vi "Image position.vi"(7 "pageNum":i32=1, 8 "error in (no error)":errorcluster, 10 "Watermark cluster IN":T1={"Show? (F)"=TRUE, "Watermark type"=enum."Text", "Opacity (%)"=100.0, "Alignment"=enum."Left", "Rotate(°)"=0.0, "Watermark"=enum."Absolute", "X (mm)"=25.0, "Y (mm)"=267.4, "Text"="", "Font"={"Name"="", "Size"=12.0, "Color"=0, "Style"={"Bold"=FALSE, "Italic"=FALSE, "Underline"=FALSE, "Strikeout"=FALSE}}, "Image path"=path "", "Image (%)"=12.0}, 11 "Image IN":refnum<k24>) -> (0 "error out":errorcluster, 2 "output cluster OUT":T1={"Show? (F)"=FALSE, "Watermark type"=enum."Text", "Opacity (%)"=10.0, "Alignment"=enum."Center", "Rotate(°)"=45.0, "Watermark"=enum."Absolute", "X (mm)"=720.0, "Y (mm)"=0.0, "Text"="", "Font"={"Name"="", "Size"=12.0, "Color"=0, "Style"={"Bold"=FALSE, "Italic"=FALSE, "Underline"=FALSE, "Strikeout"=FALSE}}, "Image path"=path "", "Image (%)"=100.0}, 3 "Image OUT":refnum<k24>)   [LabVIEW 2019]
doc: "Version 1.0\nDeveloped by Jean-Marc Simard\nCopyright © 2010, Exaprom Inc.\nAll rights reserved.\nLicense: BSD\n\nWith iTextSharp 4.1.6 (http://itextsharp.sourceforge.net)\nunder Mozilla Public License Version 1.1\n(http://www.mozilla.org/MPL/MPL-1.1.html)"
uses:
  C:/work/niobrara_lv/labview pdf writer fixing/DLL/itextsharp.dll
  DLL/itextsharp.dll
  Controls/Font Controls/Font size.ctl
  Controls/Font Controls/Font color.ctl
  Controls/Font Controls/Font cluster.ctl
  Controls/Header, Footer and Watermark Controls/Header footer horiz alignment.ctl
  <userlib>/Exaprom PDF/Controls/Watermark Page Position.ctl
  Controls/Header, Footer and Watermark Controls/Watermark cluster.ctl
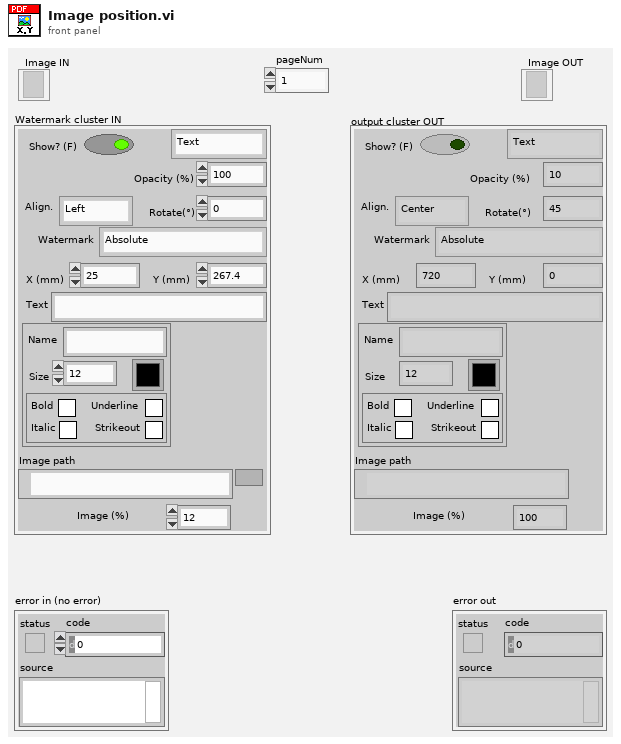
[diagram p1: front panel]
types:
  T1 = typedef "Watermark cluster.ctl" = cluster{"Show? (F)":bool, "Watermark type":enum16{"Text", "Text auto", "Image"}, "Opacity (%)":sgl, "Alignment":T2, "Rotate(°)":sgl, "Watermark":T3, "X (mm)":sgl, "Y (mm)":sgl, "Text":string, "Font":T4, "Image path":path, "Image (%)":sgl}
  T2 = typedef "Header footer horiz alignment.ctl" = enum16{"Left", "Center", "Right"}
  T3 = typedef "Watermark Page Position.ctl" = enum16{"Absolute", "Center on page", "Center on text section"}
  T4 = typedef "Font cluster.ctl" = cluster{"Name":string, "Size":T5, "Color":T6, "Style":cluster{"Bold":bool, "Italic":bool, "Underline":bool, "Strikeout":bool}}
  T5 = typedef "Font size.ctl" = sgl
  T6 = typedef "Font color.ctl" = u32
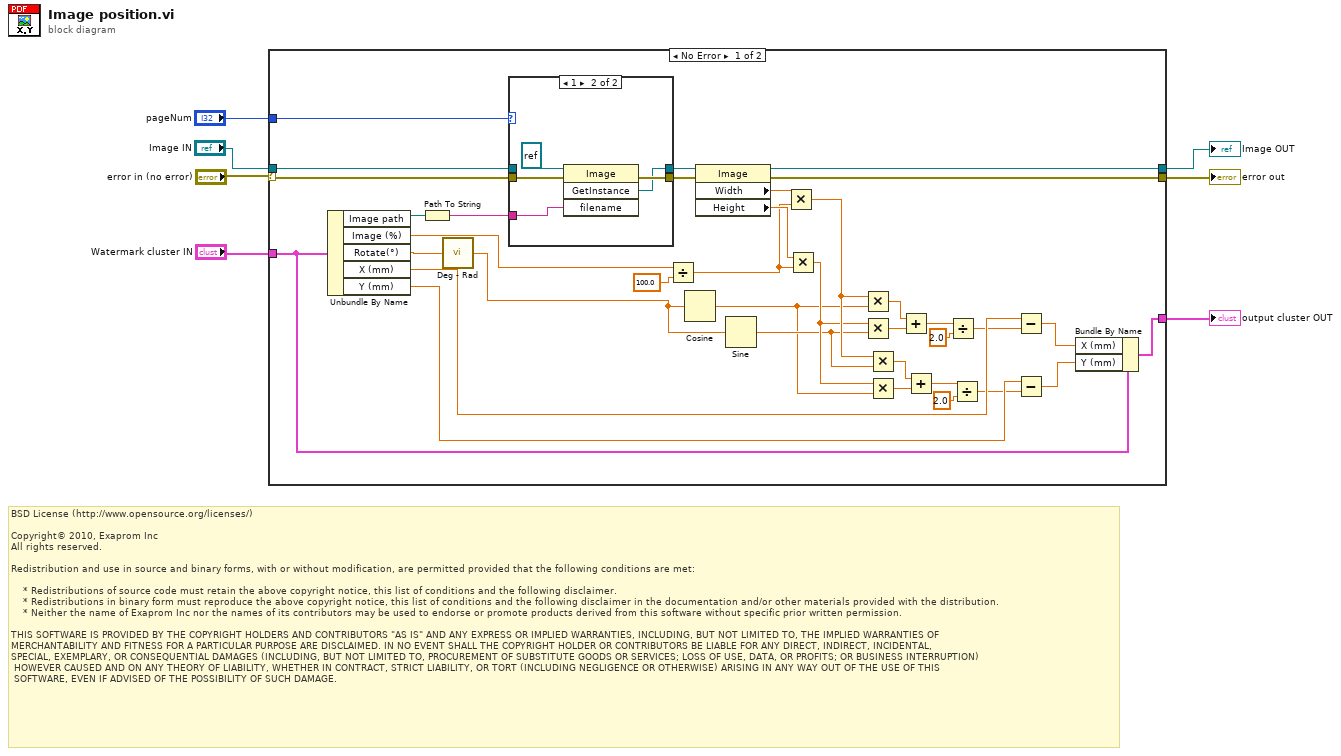
[diagram p0: block diagram]
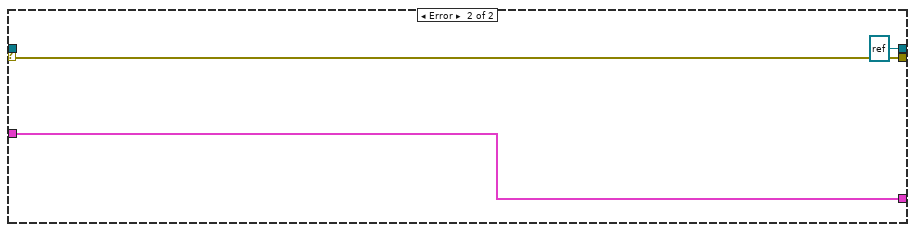
[diagram p3: hidden frame]
diagram:
  # "BSD License (http://www.opensource.org/licenses/)\n\nCopyright© 2010, Exaprom Inc\nAll rights reserved.\n\nRedistribution and use in source and binary forms, with or without modification, are permitted provided that the following conditions are met:\n\n    * Redistributions of source code must retain the above copyright notice, this list of conditions and the following disclaimer.\n    * Redistributions in binary form must reproduce the above copyright notice, this list of conditions and the following disclaimer in the documentation and/or other materials provided with the distribution.\n    * Neither the name of Exaprom Inc nor the names of its contributors may be used to endorse or promote products derived from this software without specific prior written permission.\n\nTHIS SOFTWARE IS PROVIDED BY THE COPYRIGHT HOLDERS AND CONTRIBUTORS \"AS IS\" AND ANY EXPRESS OR IMPLIED WARRANTIES, INCLUDING, BUT NOT LIMITED TO, THE IMPLIED WARRANTIES OF \nMERCHANTABILITY AND FITNESS FOR A PARTICULAR PURPOSE ARE DISCLAIMED. IN NO EVENT SHALL THE COPYRIGHT HOLDER OR CONTRIBUTORS BE LIABLE FOR ANY DIRECT, INDIRECT, INCIDENTAL,\nSPECIAL, EXEMPLARY, OR CONSEQUENTIAL DAMAGES (INCLUDING, BUT NOT LIMITED TO, PROCUREMENT OF SUBSTITUTE GOODS OR SERVICES; LOSS OF USE, DATA, OR PROFITS; OR BUSINESS INTERRUPTION)\n HOWEVER CAUSED AND ON ANY THEORY OF LIABILITY, WHETHER IN CONTRACT, STRICT LIABILITY, OR TORT (INCLUDING NEGLIGENCE OR OTHERWISE) ARISING IN ANY WAY OUT OF THE USE OF THIS\n SOFTWARE, EVEN IF ADVISED OF THE POSSIBILITY OF SUCH DAMAGE."
  n1 = case shown="No Error" "error in (no error)" {
    selector: "error in (no error)" -> [w10 w53]
    tunnel: [w39 refnum<k24> refnum ("GetInstance")] -> w3
    tunnel: [w38 w53] -> w4
    tunnel: "Watermark cluster IN" -> [w14 w51]
    tunnel: [w11 w51] -> w6
    tunnel: "pageNum" -> [w9 _]
    tunnel: "Image IN" -> [w8 _]
    frame No Error {
      n2 = Unbundle By Name(w14) -> ("Image path"=w43:path, "Image (%)"=w34:sgl, "Rotate(°)"=w37:sgl, "X (mm)"=w22:sgl, "Y (mm)"=w21:sgl)
      n3 = Path To String(path=w43) -> (string=w42:string)
      n4 = call "Deg - Rad.vi"("Degrees IN"=w37) -> ("Radian OUT"=w31:dbl)
      n5 = case shown="1" w9 {
        tunnel: w42 -> [_ w49]
        tunnel: [w44 w48] -> w41
        tunnel: [w45 w47] -> w40
        tunnel: w10 -> [w44 w46]
        tunnel: w8 -> [w45 _]
        frame 0, Default {
        }
        frame 1 {
          n6 = invoke class="Image" method="GetInstance"(reference=refnum<k24> refnum ("image"), error in=w46, "filename"=w49) -> (error out=w48:errorcluster, "GetInstance"=w47:refnum<k24>)  [unwired: 1 in, 2 out]
        }
      }
      n7 = Divide(x=w34, y=sgl 100.0) -> (x/y=w32:sgl)
      n8 = Cosine(x=w31) -> (cos(x)=w23:dbl)
      n9 = property class="Image"(reference=w40, error in=w41) -> (reference out=w39:refnum<k24>, error out=w38:errorcluster, "Width"=w36:sgl, "Height"=w35:sgl)
      n10 = Sine(x=w31) -> (sin(x)=w24:dbl)
      n11 = Multiply(x=w36, y=w32) -> (x*y=w26:sgl)
      n12 = Multiply(x=w35, y=w32) -> (x*y=w25:sgl)
      n13 = Multiply(x=w26, y=w23) -> (x*y=w30:dbl)
      n14 = Multiply(x=w25, y=w24) -> (x*y=w27:dbl)
      n15 = Multiply(x=w26, y=w24) -> (x*y=w28:dbl)
      n16 = Multiply(x=w25, y=w23) -> (x*y=w29:dbl)
      n17 = Add(x=w30, y=w27) -> (x+y=w19:dbl)
      n18 = Add(x=w28, y=w29) -> (x+y=w15:dbl)
      n19 = Divide(x=w19, y=2.0) -> (x/y=w20:dbl)
      n20 = Divide(x=w15, y=2.0) -> (x/y=w16:dbl)
      n21 = Subtract(x=w22, y=w20) -> (x-y=w13:dbl)
      n22 = Subtract(x=w21, y=w16) -> (x-y=w12:dbl)
      n23 = Bundle By Name(cluster=w14, "X (mm)"=w13, "Y (mm)"=w12) -> (w11:T1)
    }
    frame Error {
    }
  }
  "error out" <- w4
  "output cluster OUT" <- w6
  "Image OUT" <- w3
